vi "Create.vi"(8 "error in (no error)":errorcluster, 10 "Resource":refnum<visa-resource-name>, 11 "VisaResource in":refnum<class "VisaResource.lvclass">) -> (0 "error out":errorcluster, 3 "VisaResource out":refnum<class "VisaResource.lvclass">)   [LabVIEW 2020, in "PicoG-Core.lvlib" / "VisaResource.lvclass"]
uses:
  VisaResource.lvclass
  VisaResource.lvclass/VisaResource.ctl
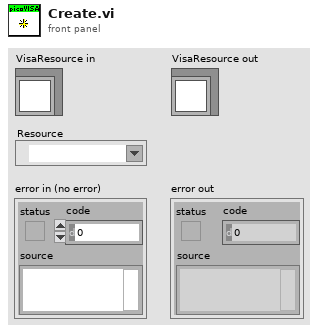
[diagram p1: front panel]
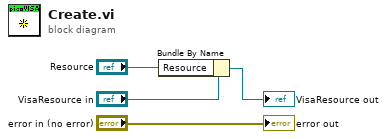
[diagram p0: block diagram]
diagram:
  n1 = Bundle By Name(cluster="VisaResource in", "Resource"="Resource") -> (→"VisaResource out":refnum<class "VisaResource.lvclass">)
  "error out" <- "error in (no error)"
